vi "call Jl server fn.vi"(8 "error in (no error)":errorcluster, 9 "binary data in":u8[](array[numeric]), 10 "JSON string in":string) -> (0 "error out":errorcluster, 1 "timeout?":bool, 2 "binary data received":u8[](array[numeric]), 3 "JSON received":string, 4 "Jl Server state out":T1, 5 "return code":u8, 6 "detailed error info":T2)   [LabVIEW 2018, in "LV-0mq-Julia_roundtrip-lib.lvlib"]
uses:
  LV-0mq-Julia_roundtrip-lib.lvlib
  detailed error info.ctl
  StackFrame.ctl
  Server or client state.ctl
  commands LV2Jl.ctl
  Commands.ctl
panel:
  out "jl stack trace":bool
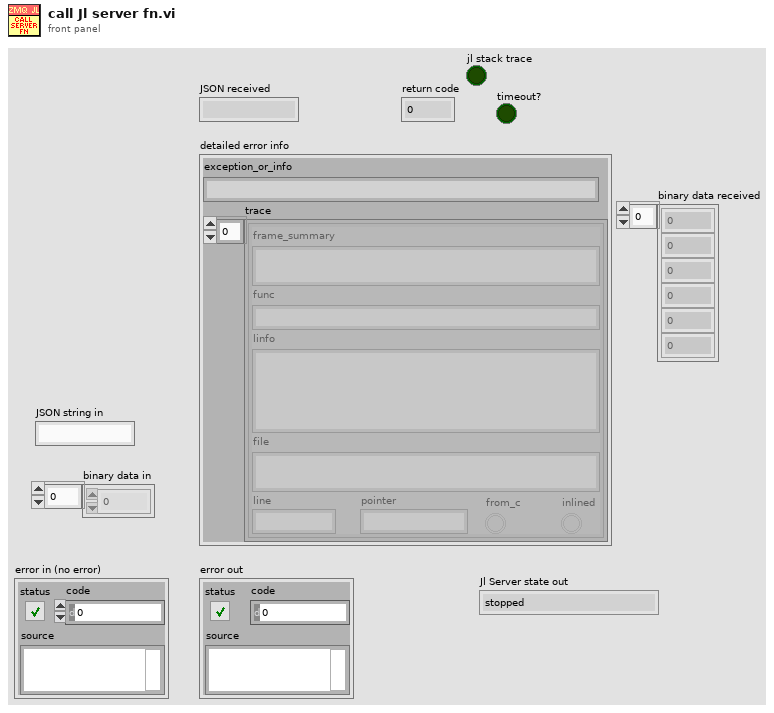
[diagram p1: front panel]
types:
  T1 = typedef "LV-0mq-Julia_roundtrip-lib.lvlib/Server or client state.ctl" = enum16{"stopped", "running", "unknown"}
  T2 = typedef "LV-0mq-Julia_roundtrip-lib.lvlib/detailed error info.ctl" = cluster{"exception_or_info":string, "trace":T3[]}
  T3 = typedef "LV-0mq-Julia_roundtrip-lib.lvlib/StackFrame.ctl" = cluster{"frame_summary":string, "func":string, "linfo":string, "file":string, "line":i32, "pointer":u64, "from_c":bool, "inlined":bool}
  T4 = typedef "LV-0mq-Julia_roundtrip-lib.lvlib/Commands.ctl" = enum16{"Start Jl-server & Init LV-client", "Send request & Get response ", "Stop Jl-server & Cleanup LV-client", "Cleanup LV-client", "Start Jl-server", "Stop Jl-server", "Init LV-Client", "Cleanup LV-Client", "(not allowed)", "Set LV Client state", "Set Jl Server state", "set ZMQ timeout", "read ZMQ timeout", "read-out state"}
  T5 = typedef "LV-0mq-Julia_roundtrip-lib.lvlib/commands LV2Jl.ctl" = u8
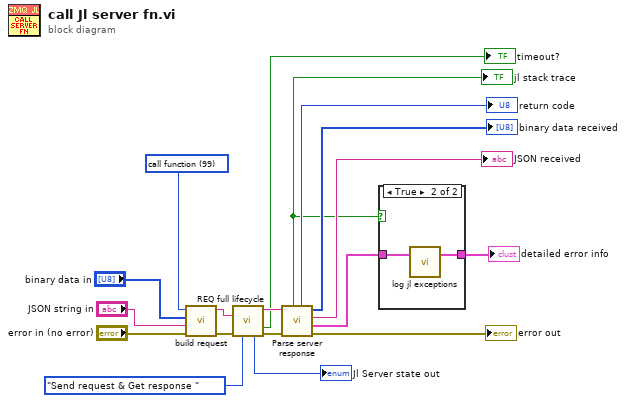
[diagram p0: block diagram]
diagram:
  w12 = T5 99 items=["call function"=99, "ping"=112, "stop"=115, "unused"=254] ("Command")
  n1 = call "build request.vi"("error in (no error)"="error in (no error)", "JSON data"="JSON string in", "binary data"="binary data in", "Command"=w12) -> ("error out"=w10:errorcluster, "REQ string"=w11:string)  [unwired: 6 in]
  n2 = call "REQ full lifecycle.vi"("data to send"=w11, "error in"=w10, "command"=Commands."Send request & Get response ") -> ("server response"=w16:string, "timeout?"=→"timeout?":bool, "Jl Server state out"=→"Jl Server state out":T1, "error out"=w15:errorcluster)  [unwired: 6 in, 3 out]
  n3 = call "Parse server response.vi"("error in (no error)"=w15, "server response in"=w16) -> ("error out"=→"error out":errorcluster, "detailed error info"=w3:T2, "JSON out"=→"JSON received":string, "binary data"=→"binary data received":u8[], "return code"=→"return code":u8, "jl stack trace"=w1:bool)  [unwired: 2 in, 2 out]
  "jl stack trace" <- w1
  n4 = case shown="True" w1 {
    tunnel: w3 -> [w19 w21]
    tunnel: [w19 w20] -> w2
    frame False {
    }
    frame True {
      n5 = call "log jl exceptions.vi"("jl error info"=w21) -> ("dup jl error info"=w20:T2)  [unwired: 2 in]
    }
  }
  "detailed error info" <- w2
